vi "TurretAnglePID.vi"(5 "TAReset":bool, 6 "TAGains":T1={"proportional gain (Kc)"=1.0, "integral time (Ti, min)"=0.01, "derivative time (Td, min)"=0.0} {"derivative time (Td, min)" format="%.3f"; "integral time (Ti, min)" format="%.3f"; "proportional gain (Kc)" format="%.3f"}, 7 "TARange":cluster{"output high":dbl, "output low":dbl}={"output high"=0.6, "output low"=-0.6} {"output low" format="%.2f"; "output high" format="%.2f"}, 8 "TADisable Range":dbl, 9 "TAIntegral Range":dbl=10000.0, 10 "TAProcess variable":dbl, 11 "TASetpoint":dbl) -> (2 "TAoutput":dbl format="%.2f")   [LabVIEW 2019]
uses:
  <vilib>/addons/control/pid/NI_PID_pid.lvlib
  <vilib>/addons/control/pid/pid.llb/PID (DBL).vi
panel:
  out "TAChart":cluster{"Setpoint":dbl, "Process variable":dbl}(graph)
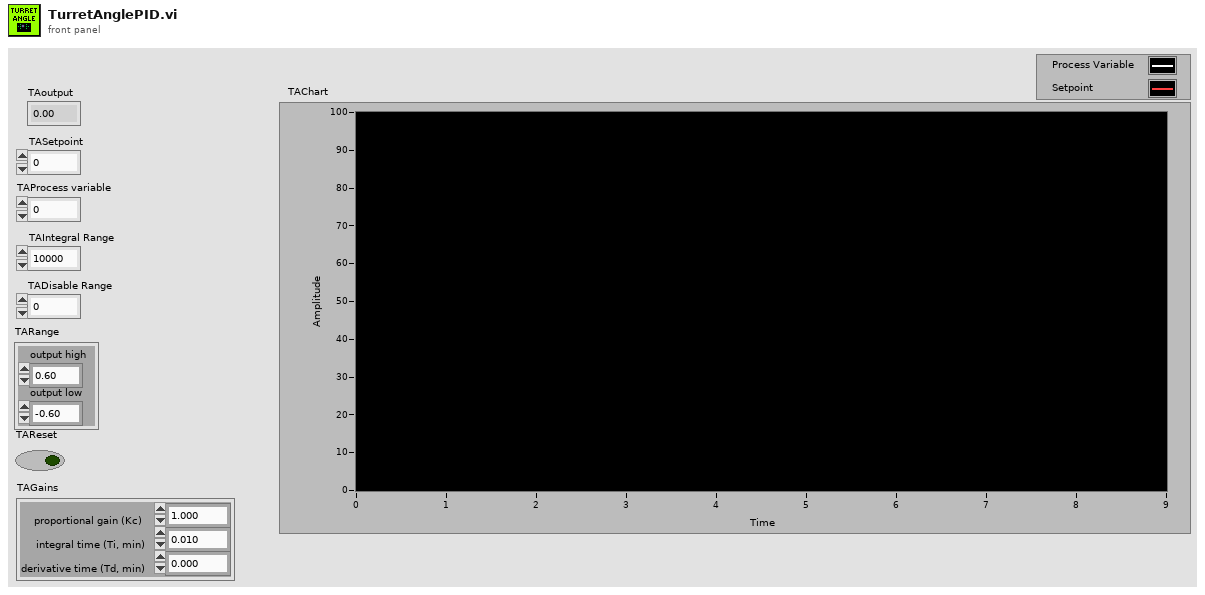
[diagram p1: front panel]
types:
  T1 = cluster{"proportional gain (Kc)":dbl, "integral time (Ti, min)":dbl, "derivative time (Td, min)":dbl}
  T2 = cluster{"TASetpoint":dbl, "TAProcess variable":dbl}
  T3 = cluster{"proportional gain (Kc)":dbl, "f":dbl, "derivative time (Td, min)":dbl}
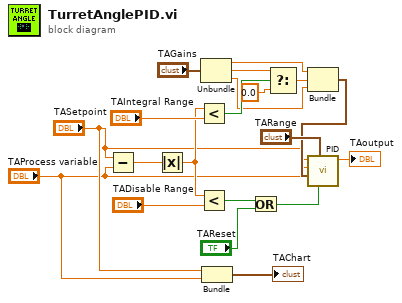
[diagram p0: block diagram]
diagram:
  n1 = Subtract(x="TASetpoint", y="TAProcess variable") -> (x-y=w19:dbl)
  n2 = Absolute Value(x=w19) -> (abs(x)=w9:dbl)
  n3 = Less?(x=w9, y="TAIntegral Range") -> (x < y?=w17:bool)
  n4 = Less?(x=w9, y="TADisable Range") -> (x < y?=w7:bool)
  n5 = Unbundle("TAGains") -> ("proportional gain (Kc)"=w12:dbl, "integral time (Ti, min)"=w15:dbl, "derivative time (Td, min)"=w11:dbl)
  n6 = Bundle("TASetpoint"="TASetpoint", "TAProcess variable"="TAProcess variable") -> (→"TAChart":T2)  [unwired: 1 in]
  n7 = Or(x=w7, y="TAReset") -> (x .or. y?=w6:bool)
  n8 = Select(t=w15, s=w17, f=0.0) -> (s? t:f=w13:dbl)
  n9 = Bundle("proportional gain (Kc)"=w12, "f"=w13, "derivative time (Td, min)"=w11) -> (w4:T3)  [unwired: 1 in]
  n10 = call-poly <vilib>:"PID.vi"("reinitialize? (F)"=w6, "output range"="TARange", "PID gains"=w4, "process variable"="TAProcess variable", "setpoint"="TASetpoint") -> ("output"=→"TAoutput":dbl)  [unwired: 5 in, 1 out]
